vi "Save_Background.vi"(9 "button":bool, 11 "averaging complete":bool) -> (1 "button on":bool, 3 "save spectrum":bool)   [LabVIEW 2013]
panel:
  in  "count":i8
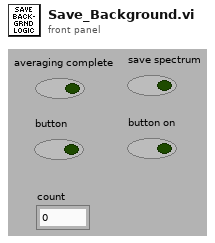
[diagram p1: front panel]
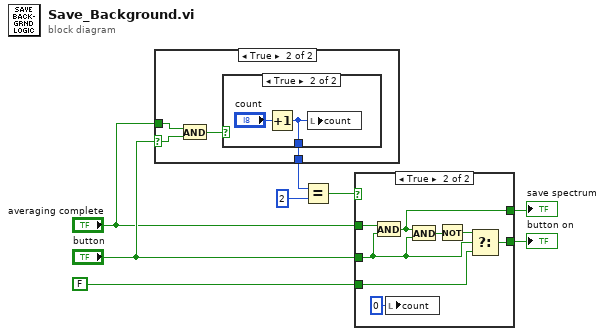
[diagram p0: block diagram]
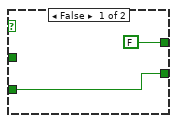
[diagram p2: hidden frame]
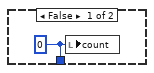
[diagram p3: hidden frame]
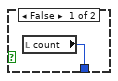
[diagram p4: hidden frame]
diagram:
  n1 = case shown="True" "button" {
    selector: "button" -> [_ w11]
    tunnel: [w9 w13] -> w4
    tunnel: "averaging complete" -> [_ w12]
    frame False {
      w9 = i8 0
      n2 = local write "count"(w9) -> ()
    }
    frame True {
      n3 = And(x=w12, y=w11) -> (x .and. y?=w10:bool)
      n4 = case shown="True" w10 {
        tunnel: [w14 w15] -> w13
        frame False {
          n5 = local read "count"() -> (w14:i8)
        }
        frame True {
          n6 = Increment(x="count") -> (x+1=w15:i8)
          n7 = local write "count"(w15) -> ()
        }
      }
    }
  }
  n8 = Equal?(x=w4, y=i8 2) -> (x = y?=w5:bool)
  n9 = case shown="True" w5 {
    tunnel: FALSE ("f") -> [_ w24]
    tunnel: "button" -> [w17 w23]
    tunnel: [w17 w22] -> w7
    tunnel: [FALSE w21] -> w6
    tunnel: "averaging complete" -> [_ w20]
    frame False {
    }
    frame True {
      n10 = And(x=w20, y=w23) -> (x .and. y?=w21:bool)
      n11 = local write "count"(i8 0) -> ()
      n12 = And(x=w21, y=w23) -> (x .and. y?=w26:bool)
      n13 = Not(x=w26) -> (.not. x?=w25:bool)
      n14 = Select(t=w25, s=w23, f=w24) -> (s? t:f=w22:bool)
    }
  }
  "save spectrum" <- w6
  "button on" <- w7
